vi "Plot Colormap.vi"(4 "Colormap Config":T1, 6 "Y":dbl[](array[numeric])=[0.0, 2.0, 4.0, 6.0, 8.0], 7 "target path":path=path "C:/Users/bogum/OneDrive/Dokumenty/Git/LabVIEW Python Ploter/LabVIEW_python_ploter.py", 8 "error in (no error)":errorcluster, 9 "X":dbl[](array[numeric])=[0.0, 1.0, 2.0, 3.0, 4.0], 10 "Data 2d":dbl[][](array[numeric])=[[0.0, 0.0, 2.0, 0.0, 0.0], [0.0, 1.0, 1.0, 1.0, 0.0], [1.0, 0.0, 1.0, 0.0, 1.0], [0.0, 0.0, 1.0, 0.0, 0.0], [0.0, 0.0, 1.0, 0.0, 0.0]], 11 "PythonPlotter in":refnum<class "PythonPlotter.lvclass">) -> (0 "error out":errorcluster, 3 "PythonPlotter out":refnum<class "PythonPlotter.lvclass">)   [LabVIEW 2024, in "PythonPlotter.lvclass"]
uses:
  PythonPlotter.lvclass
  #ColormapConfig.ctl
  PythonPlotter.lvclass/PythonPlotter.ctl
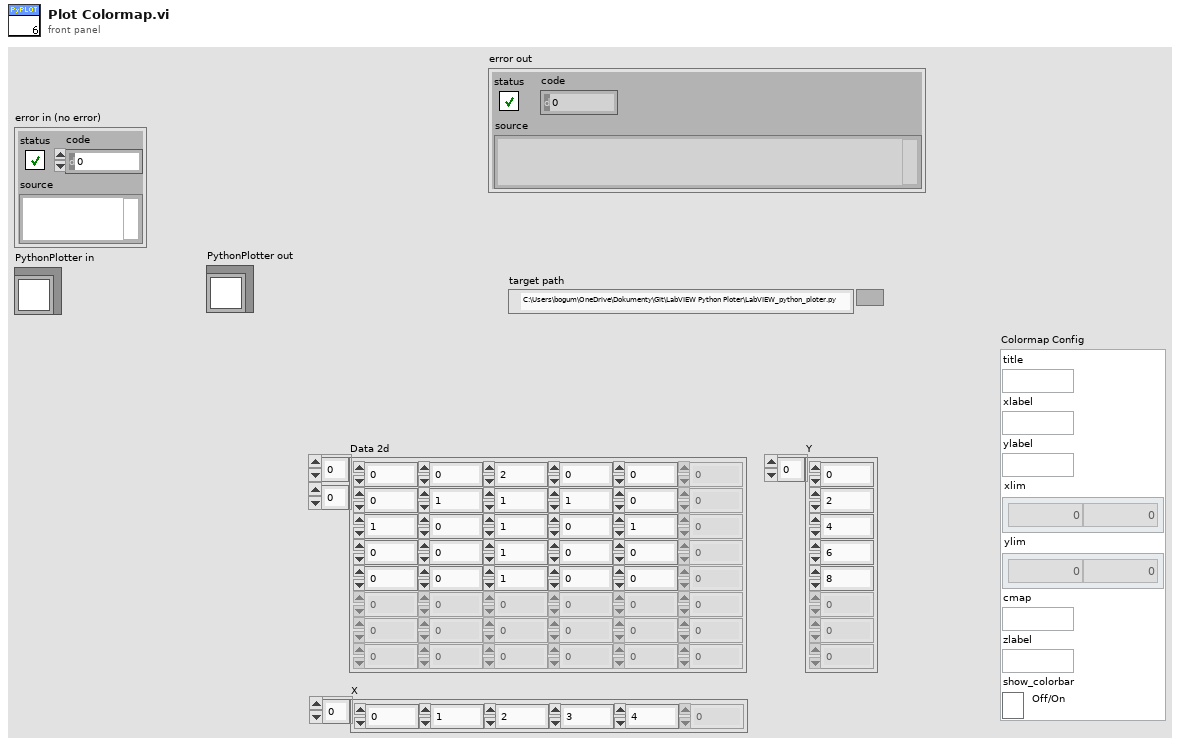
[diagram p1: front panel]
types:
  T1 = typedef "PythonPlotter.lvclass/#ColormapConfig.ctl" = cluster{"title":string, "xlabel":string, "ylabel":string, "xlim":dbl[], "ylim":dbl[], "cmap":string, "zlabel":string, "show_colorbar":bool}
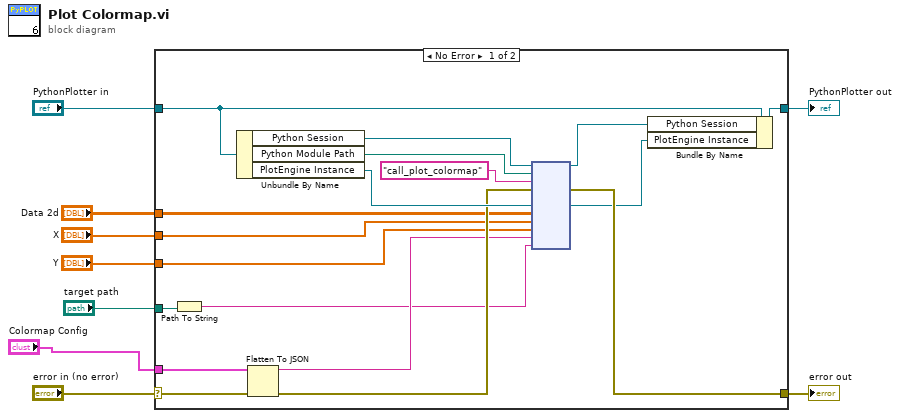
[diagram p0: block diagram]
diagram:
  n1 = case shown="No Error" "error in (no error)" {
    selector: "error in (no error)" -> [w21 w29]
    tunnel: [w16 w29] -> w8
    tunnel: [w15 w28] -> w6
    tunnel: "PythonPlotter in" -> [w27 w28]
    tunnel: "Colormap Config" -> [w22 _]
    tunnel: "Data 2d" -> [w19 _]
    tunnel: "X" -> [w18 _]
    tunnel: "target path" -> [w17 _]
    tunnel: "Y" -> [w12 _]
    frame No Error {
      n2 = Path To String(path=w17) -> (string=w10:string)
      n3 = Unbundle By Name(w27) -> ("Python Session"=w25:refnum<k35>, "Python Module Path"=w24:path, "PlotEngine Instance"=w23:refnum<k38>)
      n4 = Flatten To JSON(anything=w22, error in (no error)=w21) -> (JSON string=w11:string, 11:w20:errorcluster)  [unwired: 1 in]
      n5 = node(w25, w24, "call_plot_colormap" ("function name"), w20, w23, w19, w18, w12, w11, w10) -> (w14:refnum<k35>, w16:errorcluster, w13:refnum<k38>)  [unwired: 7 in, 2 out]
      n6 = Bundle By Name(cluster=w27, "Python Session"=w14, "PlotEngine Instance"=w13) -> (w15:refnum<class "PythonPlotter.lvclass">)
    }
    frame Error {
    }
  }
  "error out" <- w8
  "PythonPlotter out" <- w6
